vi "ControlTEST_V1.vi"(4 "Días entre TEST 2":i16(slide) scale=0.0..50.0, 5 "Ultimo TEST":timestamp, 6 "Horario TEST":string) -> (2 "Boolean":bool)   [LabVIEW 2015]
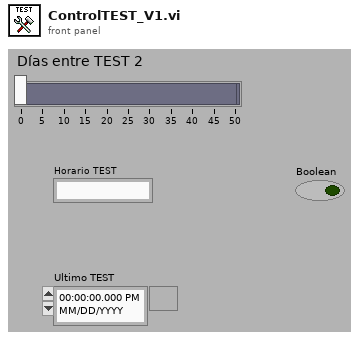
[diagram p1: front panel]
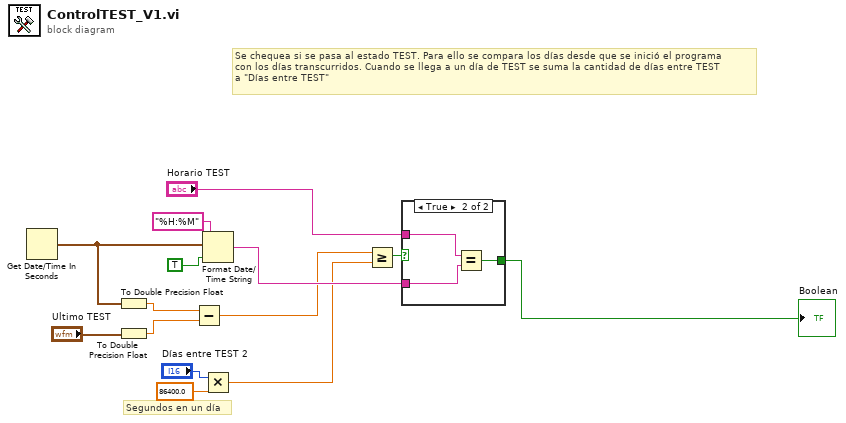
[diagram p0: block diagram]
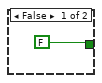
[diagram p2: hidden frame]
diagram:
  # "Segundos en un día"
  # "Se chequea si se pasa al estado TEST. Para ello se compara los días desde que se inició el programa\ncon los días transcurridos. Cuando se llega a un día de TEST se suma la cantidad de días entre TEST\na \"Días entre TEST\""
  n1 = Get Date/Time In Seconds() -> (seconds since 1Jan1904=w9:timestamp)
  n2 = To Double Precision Float(number=w9) -> (double precision float=w4:dbl)
  n3 = To Double Precision Float(number="Ultimo TEST") -> (double precision float=w3:dbl)
  n4 = Subtract(x=w4, y=w3) -> (x-y=w2:dbl)
  n5 = Format Date/Time String(time format string (%c)="%H:%M", seconds (now)=w9, UTC format=TRUE) -> (date/time string=w7:string)
  n6 = Multiply(x="Días entre TEST 2", y=86400.0) -> (x*y=w1:dbl)
  n7 = Greater Or Equal?(x=w2, y=w1) -> (x >= y?=w13:bool)
  n8 = case shown="True" w13 {
    tunnel: w7 -> [_ w18]
    tunnel: [FALSE w17] -> w14
    tunnel: "Horario TEST" -> [_ w16]
    frame False {
    }
    frame True {
      n9 = Equal?(x=w16, y=w18) -> (x = y?=w17:bool)
    }
  }
  "Boolean" <- w14
